vi "Step Simulation.vi"(0 "reference in":refnum<class "Battery.lvclass">, 1 "current_A":dbl=1.0, 2 "time_step_S":dbl=0.0015 format="%#_13g", 5 "Error In":errorcluster) -> (14 "reference out":refnum<class "Battery.lvclass">, 15 "terminal_voltage_V":dbl, 19 "Error Out":errorcluster)   [LabVIEW 2023, in "Battery.lvclass"]
uses:
  Battery.lvclass
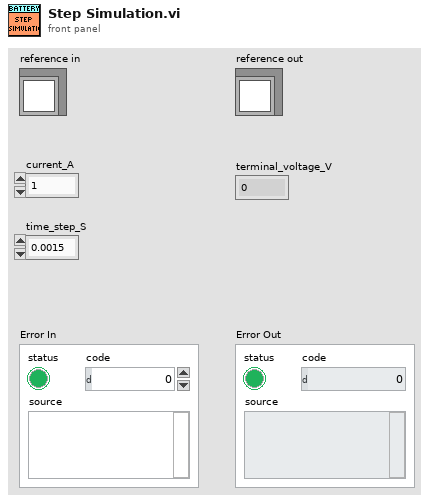
[diagram p1: front panel]
types:
  T1 = typedef "Battery.lvclass/ObjectAttributes.ctl" = cluster{"Python module":path, "Python Session":refnum<k35>, "PybammWrapper":refnum<k38>, "model loaded":bool, "simulation loaded":bool}
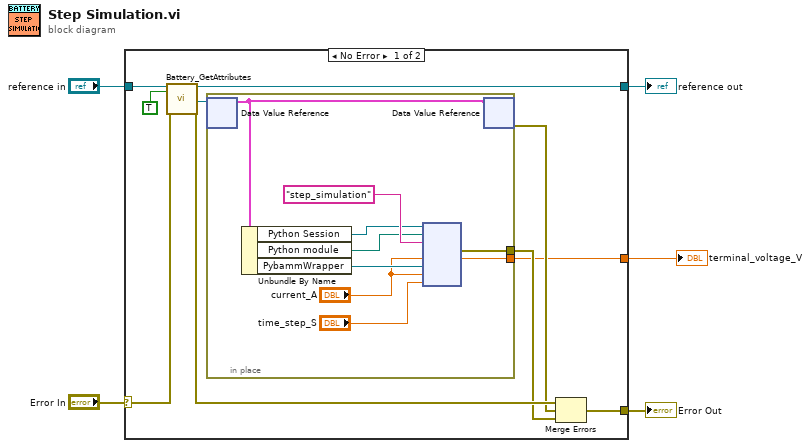
[diagram p0: block diagram]
diagram:
  n1 = case shown="No Error" "Error In" {
    selector: "Error In" -> [w14 w26]
    tunnel: [w12 w26] -> w4
    tunnel: [w13 w25] -> w2
    tunnel: "reference in" -> [w15 w25]
    tunnel: [w6 _] -> w1
    frame No Error {
      n2 = call "Battery_GetAttributes.vi"("reference in"=w15, "OnlyGetDvrReference(False)"=TRUE, "Error In"=w14) -> ("reference out"=w13:refnum<class "Battery.lvclass">, "DataRef"=w11:refnum<data-value>, "Error Out"=w9:errorcluster)  [unwired: 13 in, 1 out]
      n3 = in-place {
        in-place-border: [w23] -> w7
        in-place-border: [w16] -> w6
        n4 = in-place-dvr #1(w11) -> (w18:T1)  [unwired: 1 out]
        n5 = Unbundle By Name(w18) -> ("Python Session"=w20:refnum<k35>, "Python module"=w21:path, "PybammWrapper"=w22:refnum<k38>)
        n6 = node(w20, w21, "step_simulation" ("function name"), "current_A", w22, "current_A", "time_step_S") -> (w23:errorcluster, w16:dbl)  [unwired: 4 in, 3 out]
        n7 = in-place-dvr #1(w18) -> (w8:errorcluster)  [unwired: 1 out]
      }
      n8 = Merge Errors(w9, w8, w7) -> (w12:errorcluster)
    }
    frame Error {
    }
  }
  "Error Out" <- w4
  "reference out" <- w2
  "terminal_voltage_V" <- w1
